vi "Release All Events.vi"(8 "error in (no error)":errorcluster, 11 "Events":T1) -> (0 "error out":errorcluster)   [LabVIEW 2023, in "HAF.lvlib"]
doc: "Destroys all Event references making them invalid."
uses:
  HAF.lvlib
  Event Data.ctl
  Stop Event.ctl
  Pause Event.ctl
  Resume Event.ctl
  Done Event.ctl
  All Events.ctl
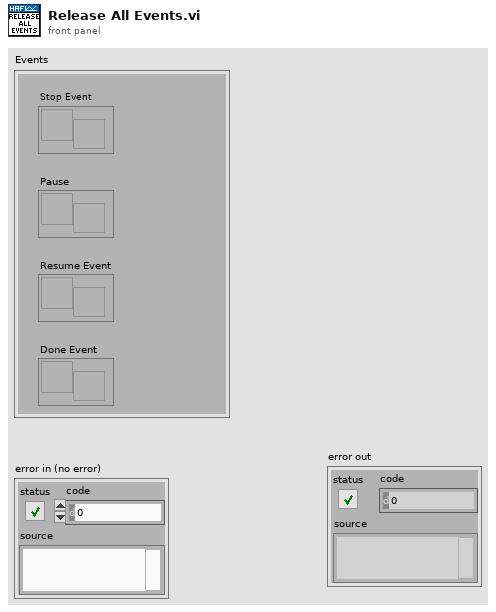
[diagram p1: front panel]
types:
  T1 = typedef "HAF.lvlib/All Events.ctl" = cluster{"Stop Event":T2, "Pause":T3, "Resume Event":T4, "Done Event":T5}
  T2 = typedef "HAF.lvlib/Stop Event.ctl" = refnum<user-event>
  T3 = typedef "HAF.lvlib/Pause Event.ctl" = refnum<user-event>
  T4 = typedef "HAF.lvlib/Resume Event.ctl" = refnum<user-event>
  T5 = typedef "HAF.lvlib/Done Event.ctl" = refnum<user-event>
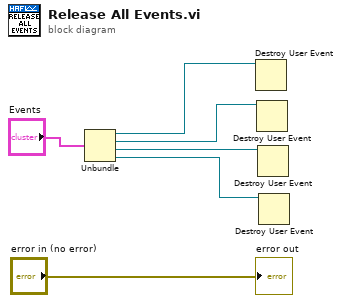
[diagram p0: block diagram]
diagram:
  n1 = Unbundle("Events") -> ("Stop Event"=w5:T2, "Pause"=w4:T3, "Resume Event"=w3:T4, "Done Event"=w2:T5)
  n2 = Destroy User Event(user event=w5) -> ()  [unwired: 1 in, 1 out]
  n3 = Destroy User Event(user event=w4) -> ()  [unwired: 1 in, 1 out]
  n4 = Destroy User Event(user event=w3) -> ()  [unwired: 1 in, 1 out]
  n5 = Destroy User Event(user event=w2) -> ()  [unwired: 1 in, 1 out]
  "error out" <- "error in (no error)"
